vi "Write State Name.vi"(8 "error in (no error)":errorcluster, 10 "State Name":string, 11 "Command States in":refnum<class "Command States.lvclass">) -> (0 "error out":errorcluster, 3 "Command States out":refnum<class "Command States.lvclass">)   [LabVIEW 2013, in "Command Actor.lvlib" / "Command States.lvclass"]
uses:
  Command States.lvclass
  Command States.lvclass/Command States.ctl
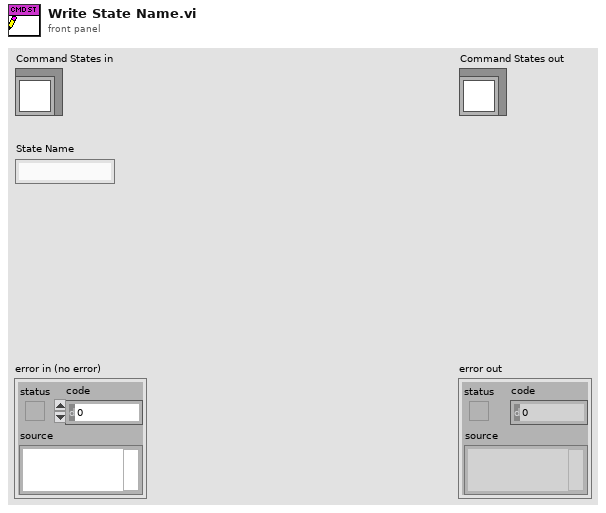
[diagram p1: front panel]
types:
  T1 = typedef "Command Actor.lvlib/Command States.lvclass/State Status.ctl" = cluster{"State Name":string, "State Entry Time":timestamp, "State Exit Time":timestamp}
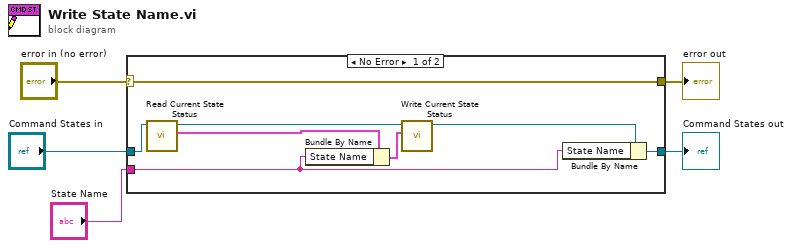
[diagram p0: block diagram]
diagram:
  n1 = case shown="No Error" "error in (no error)" {
    selector: "error in (no error)" -> [w13 w15]
    tunnel: [w13 w15] -> w4
    tunnel: "State Name" -> [w8 _]
    tunnel: "Command States in" -> [w11 w14]
    tunnel: [w6 w14] -> w1
    frame No Error {
      n2 = call-dynamic "Read Current State Status.vi"("Command States in"=w11) -> ("State Status"=w10:T1, "Command States out"=w12:refnum<class "Command States.lvclass">)  [unwired: 8 in, 1 out]
      n3 = Bundle By Name(cluster=w10, "State Name"=w8) -> (w9:T1)
      n4 = call-dynamic "Write Current State Status.vi"("State Status"=w9, "Command States in"=w12) -> ("Command States out"=w7:refnum<class "Command States.lvclass">)  [unwired: 8 in, 1 out]
      n5 = Bundle By Name(cluster=w7, "State Name"=w8) -> (w6:refnum<class "Command States.lvclass">)
    }
    frame Error {
    }
  }
  "error out" <- w4
  "Command States out" <- w1
